vi "Configure Echo Gate Parameters.vi"(7 "Micropulse # In":i32, 8 "error in (no error)":errorcluster, 9 "Echo Gate Parameters":T2={"Start (us)"=0.0, "Length (us)"=0.0, "Threshold"=10, "Colour"=0} {"Threshold" min=10 max=4095 step=10; "Length (us)" min=0.0 max=96000.0 step=100.0; "Start (us)" min=0.0 max=64000.0 step=100.0}, 10 "Echo Trigger Mode":T1, 11 "Test Number":u32) -> (0 "error out":errorcluster, 3 "Test Number Out":u32, 5 "Micropulse # Out":i32)   [LabVIEW 2026, in "MicroPulse_Driver.lvlib"]
uses:
  MicroPulse_Driver.lvlib
  Data/Datatypes/MP - echo gate parameters.ctl
  Data/Datatypes/MP - echo gate mode.ctl
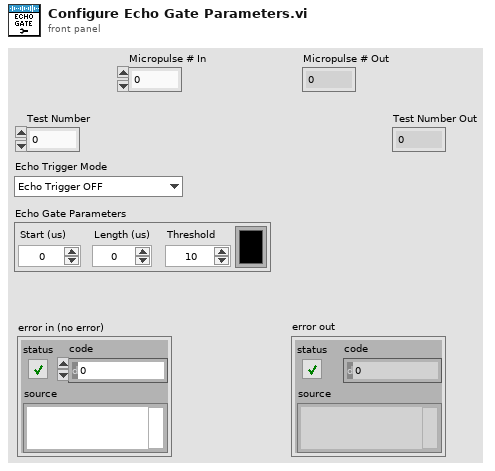
[diagram p1: front panel]
types:
  T1 = typedef "MicroPulse_Driver.lvlib/MP - echo gate mode.ctl" = enum16{"Echo Trigger OFF", "Echo Gate Display Mode", "Echo Trigger ON", "Multi Gate or FMC Mode", "Reserved", "PA - Echo Trigger ON"}
  T2 = typedef "MicroPulse_Driver.lvlib/MP - echo gate parameters.ctl" = cluster{"Start (us)":dbl, "Length (us)":dbl, "Threshold":u16, "Colour":u32}
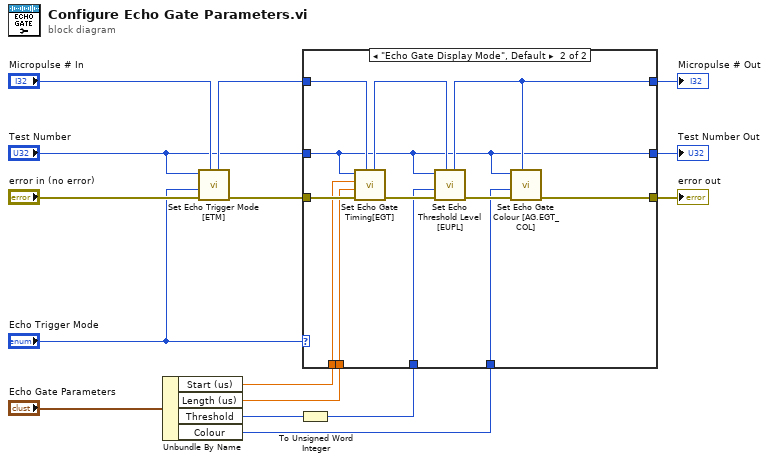
[diagram p0: block diagram]
diagram:
  n1 = Unbundle By Name("Echo Gate Parameters") -> ("Start (us)"=w8:dbl, "Length (us)"=w7:dbl, "Threshold"=w6:u16, "Colour"=w1:u32)
  n2 = call "Set Echo Trigger Mode [ETM].vi"("Micropulse # In"="Micropulse # In", "error in (no error)"="error in (no error)", "ETM Mode"="Echo Trigger Mode", "Test Number"="Test Number") -> ("error out"=w13:errorcluster, "Micropulse # Out"=w10:i32)  [unwired: 6 in]
  n3 = To Unsigned Word Integer(number=w6) -> (unsigned 16bit integer=w5:u16)
  n4 = case shown="\"Echo Gate Display Mode\", Default" "Echo Trigger Mode" {
    tunnel: [w18 w20] -> w14
    tunnel: w13 -> [w17 w29]
    tunnel: w10 -> [w18 w28]
    tunnel: [w17 w22] -> w9
    tunnel: "Test Number" -> [w16 w19]
    tunnel: w8 -> [_ w26]
    tunnel: w7 -> [_ w25]
    tunnel: w5 -> [_ w24]
    tunnel: [w16 w19] -> w2
    tunnel: w1 -> [_ w21]
    frame "Echo Trigger OFF" {
      # "#TODO\nremove EGT and EUPL commands\nfrom the command list."
    }
    frame "Echo Gate Display Mode", Default {
      n5 = call "Set Echo Gate Timing[EGT].vi"("Micropulse # In"=w28, "error in (no error)"=w29, "Gate Length (us)"=w25, "Gate Start (us)"=w26, "Test Number"=w19) -> ("error out"=w30:errorcluster, "Micropulse # Out"=w27:i32)  [unwired: 5 in]
      n6 = call "Set Echo Threshold Level [EUPL].vi"("Micropulse # In"=w27, "error in (no error)"=w30, "Threshold"=w24, "Test Number"=w19) -> ("error out"=w23:errorcluster, "Micropulse # Out"=w20:i32)  [unwired: 6 in]
      n7 = call "Set Echo Gate Colour [AG.EGT_COL].vi"("Micropulse # In"=w20, "error in (no error)"=w23, "Colour"=w21, "Test Number"=w19) -> ("error out"=w22:errorcluster)  [unwired: 6 in, 1 out]
    }
  }
  "Micropulse # Out" <- w14
  "error out" <- w9
  "Test Number Out" <- w2
